vi "Read Data.vi"(8 "error in (no error)":errorcluster, 11 "Generic Update Data Message in":refnum<class "Generic Update Data Message.lvclass">) -> (0 "error out":errorcluster, 2 "Base Data Lib:Data":refnum<class "Data.lvclass">, 3 "Generic Update Data Message out":refnum<class "Generic Update Data Message.lvclass">)   [LabVIEW 2015, in "DAQ Device.lvlib" / "Generic Update Data Message.lvclass"]
uses:
  Generic Update Data Message.lvclass
  <vilib>/MSR Consulting, LLC/General Reuse/Data/Data.lvclass
  Generic Update Data Message.lvclass/Generic Update Data Message.ctl
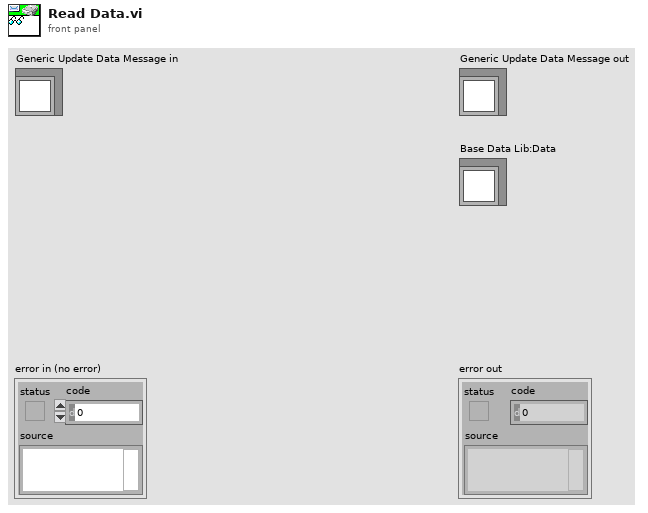
[diagram p1: front panel]
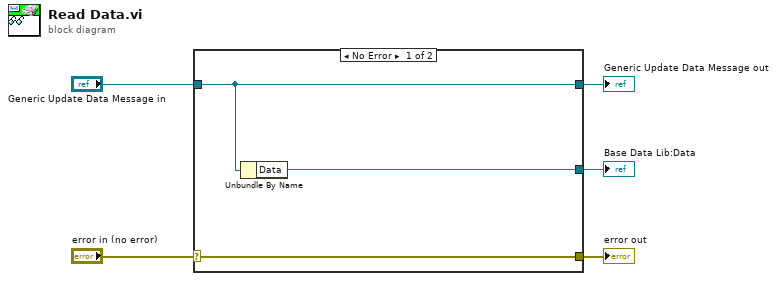
[diagram p0: block diagram]
diagram:
  n1 = case shown="No Error" "error in (no error)" {
    selector: "error in (no error)" -> [w8 w9]
    tunnel: [w8 w9] -> w4
    tunnel: [w7 w10] -> w2
    tunnel: "Generic Update Data Message in" -> [w7 w10]
    tunnel: [w6 _] -> w1
    frame No Error {
      n2 = Unbundle By Name(w7) -> ("Data"=w6:refnum<class "Data.lvclass">)
    }
    frame Error {
    }
  }
  "error out" <- w4
  "Generic Update Data Message out" <- w2
  "Base Data Lib:Data" <- w1
